vi "Create notifiers.vi"(8 "error in":errorcluster) -> (0 "error out":errorcluster, 3 "output cluster":T1)   [LabVIEW 2015]
uses:
  Notifiers.ctl
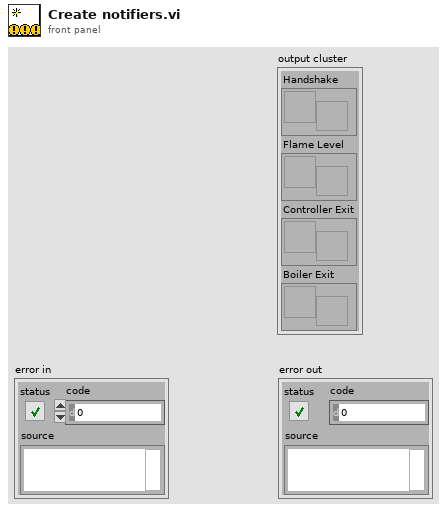
[diagram p1: front panel]
types:
  T1 = typedef "Notifiers.ctl" = cluster{"Handshake":refnum<notifier>, "Flame Level":refnum<notifier>, "Controller Exit":refnum<notifier>, "Boiler Exit":refnum<notifier>}
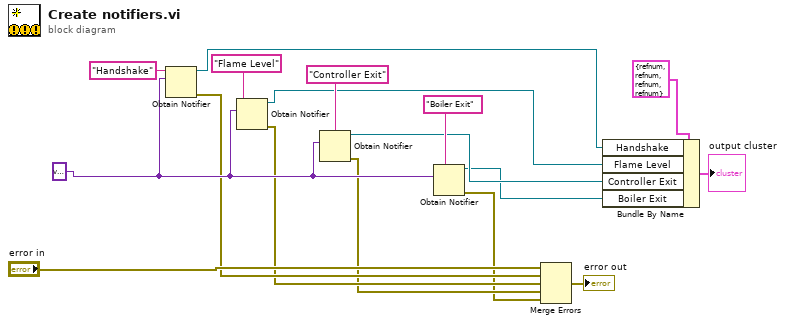
[diagram p0: block diagram]
diagram:
  w13 = variant
  n1 = Obtain Notifier(name (unnamed)="Handshake", notification data type=w13) -> (notifier out=w5:refnum<notifier>, error out=w11:errorcluster)  [unwired: 2 in, 1 out]
  n2 = Obtain Notifier(name (unnamed)="Flame Level", notification data type=w13) -> (notifier out=w4:refnum<notifier>, error out=w10:errorcluster)  [unwired: 2 in, 1 out]
  n3 = Obtain Notifier(name (unnamed)="Controller Exit", notification data type=w13) -> (notifier out=w3:refnum<notifier>, error out=w9:errorcluster)  [unwired: 2 in, 1 out]
  n4 = Obtain Notifier(name (unnamed)="Boiler Exit", notification data type=w13) -> (notifier out=w2:refnum<notifier>, error out=w8:errorcluster)  [unwired: 2 in, 1 out]
  n5 = Merge Errors("error in", w11, w10, w9, w8) -> (→"error out":errorcluster)
  n6 = Bundle By Name(cluster=T1 {"Handshake"=refnum, "Flame Level"=refnum, "Controller Exit"=refnum, "Boiler Exit"=refnum}, "Handshake"=w5, "Flame Level"=w4, "Controller Exit"=w3, "Boiler Exit"=w2) -> (→"output cluster":T1)
